vi "Step5_0_LowPass.vi"(9 "s_axis_data_tdata":fxp<+/-,24,1>, 10 "s_axis_data_tvalid":bool) -> (1 "m_axis_data_tdata":fxp<+/-,24,1>, 2 "m_axis_data_tvalid":bool, 3 "s_axis_data_tready":bool)   [LabVIEW 2018]
uses:
  <vilib>/rvi/IPIntegrationNode/IPINode_Typedef/niFpgaIPINodeSupportedFamilies.ctl
  <vilib>/rvi/IPIntegrationNode/IPINode_Utilities/niFpgaIPINodeSimCore.vi
  <vilib>/rvi/XilinxIP/XIPIN_XNode/niFpgaXIPIN.xnode
  FIR_Filter_Configuration/FIR Compiler/xsim.dir/FIR_Compiler_3CE652926F5B43F18022D1349C670FA0/xsimk_3CE652926F5B43F18022D1349C670FA0.dll
  <vilib>/rvi/IPIntegrationNode/IPINode_Xnode/niFpgaIPINode.xnode
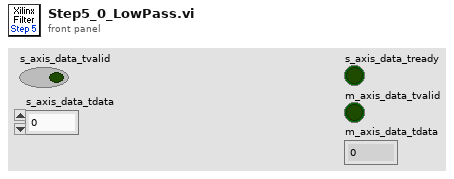
[diagram p1: front panel]
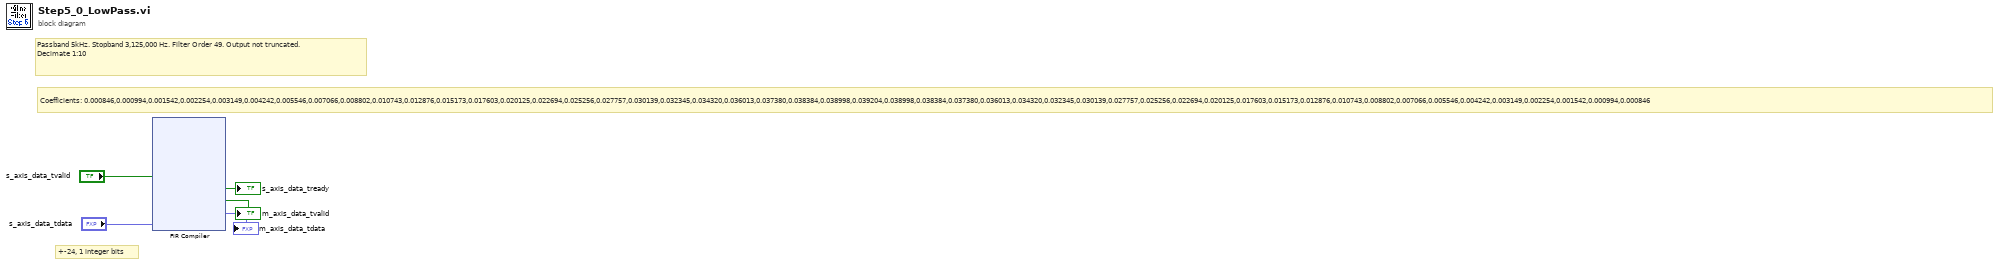
[diagram p0: block diagram]
diagram:
  # "+-24, 1 integer bits"
  # "Coefficients: 0.000846,0.000994,0.001542,0.002254,0.003149,0.004242,0.005546,0.007066,0.008802,0.010743,0.012876,0.015173,0.017603,0.020125,0.022694,0.025256,0.027757,0.030139,0.032345,0.034320,0.036013,0.037380,0.038384,0.038998,0.039204,0.038998,0.038384,0.037380,0.036013,0.034320,0.032345,0.030139,0.027757,0.025256,0.022694,0.020125,0.017603,0.015173,0.012876,0.010743,0.008802,0.007066,0.005546,0.004242,0.003149,0.002254,0.001542,0.000994,0.000846"
  # "Passband 5kHz. Stopband 3,125,000 Hz. Filter Order 49. Output not truncated.\nDecimate 1:10"
  n1 = xnode ("FIR Compiler")("s_axis_data_tvalid"="s_axis_data_tvalid", "s_axis_data_tdata"="s_axis_data_tdata") -> ("s_axis_data_tready"=→"s_axis_data_tready":bool, "m_axis_data_tvalid"=→"m_axis_data_tvalid":bool, "m_axis_data_tdata"=→"m_axis_data_tdata":fxp<+/-,24,1>)
